vi "Phase_unwrapping2.vi"(10 "Phase at Peaks":dbl[](array[numeric])=[0.5, 1.55, 1.5, -0.641593, 0.358407, 0.358407], 11 "Peak Locations":dbl[](array[numeric])=[0.0, 2.0, 3.0, 4.0]) -> ()   [LabVIEW 2016]
panel:
  out "Array 3":dbl[](array[numeric])
  out "Numeric":i32
  out "Phase out":dbl[](array[numeric])
  out "Boolean":bool
  out "Array 2":dbl[](array[numeric])
  out "Numeric 2":i32
  out "Array":dbl[](array[numeric])
  out "element":i32
  out "Missing Peaks":i32[](array[numeric])=[3, 4, 7, 8, 9]
  in  "Width":dbl=0.02 format="%#_13g"
  in  "Average Spacing":dbl=1.0 format="%#_13g"
  in  "Approximate Phase Difference":dbl=0.5 format="%#_13g"
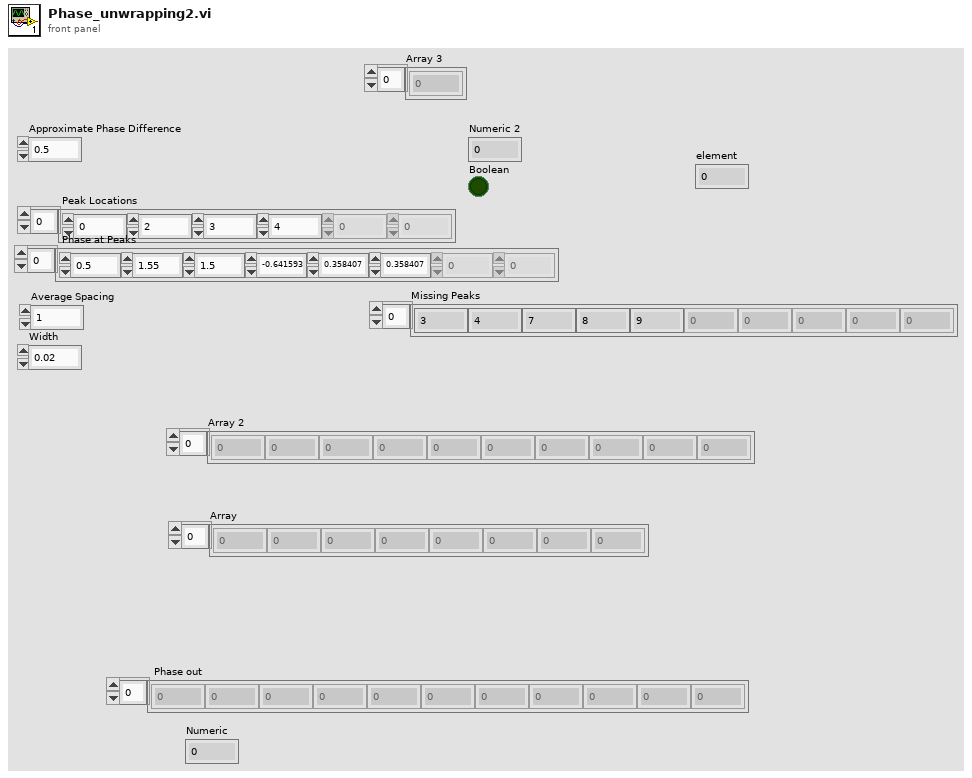
[diagram p1: front panel]
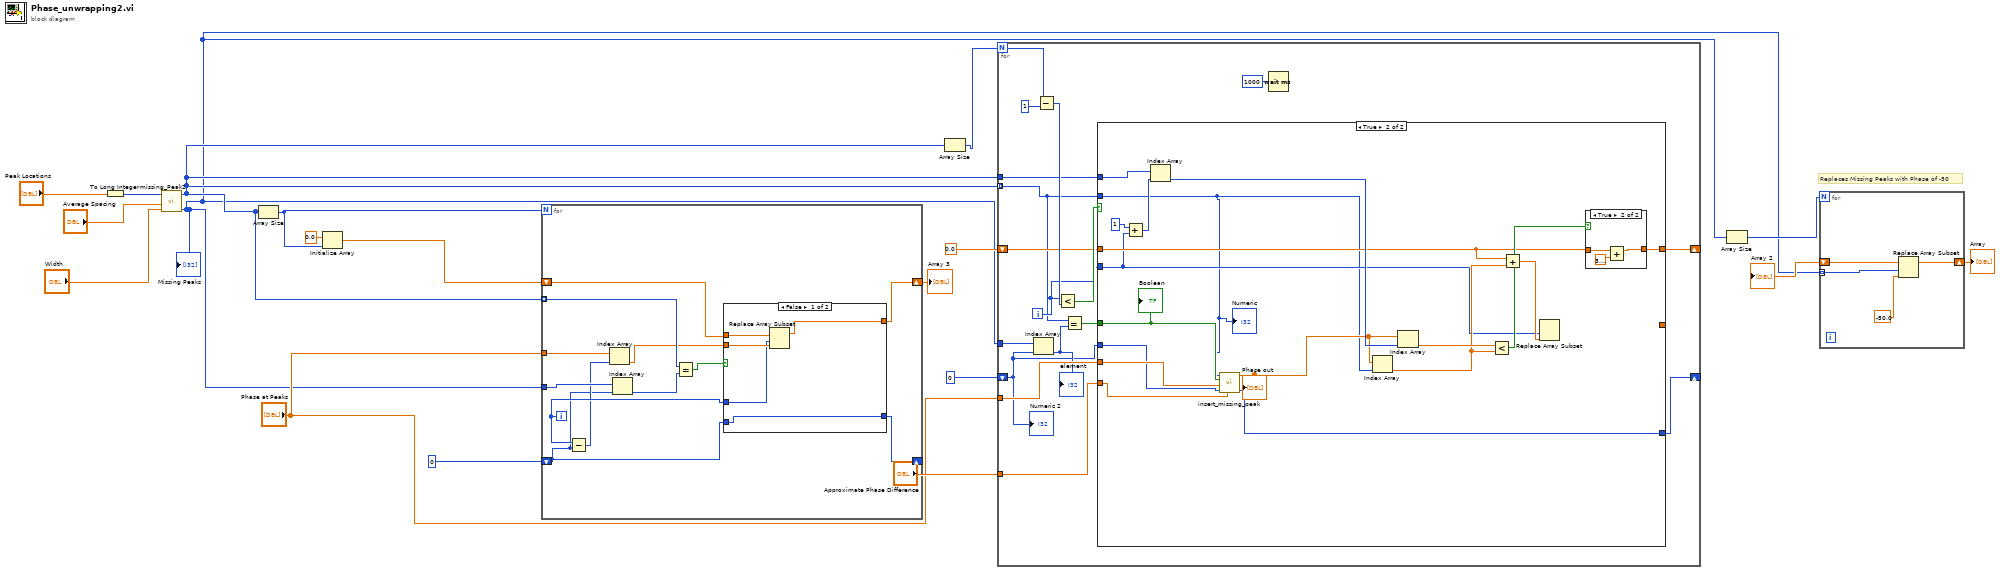
[diagram p0: block diagram]
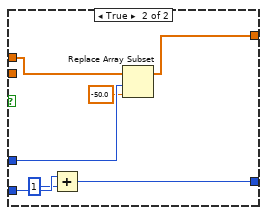
[diagram p2: hidden frame]
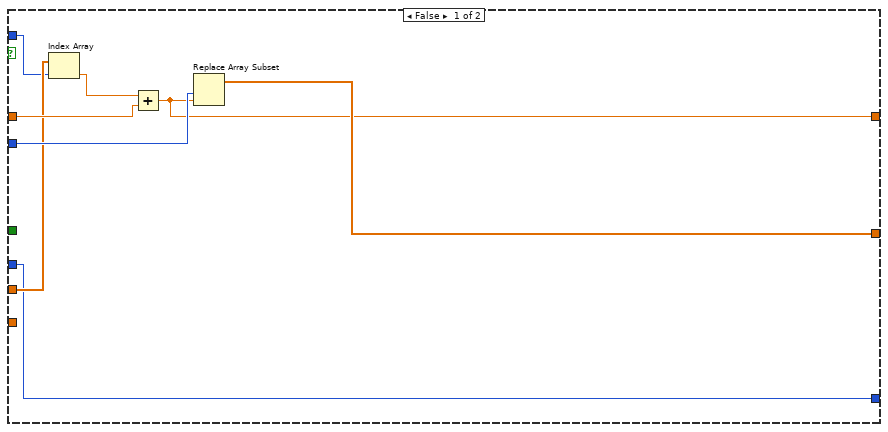
[diagram p3: hidden frame]
diagram:
  # "Replaces Missing Peaks with Phase of -50"
  n1 = To Long Integer(number="Peak Locations") -> (32bit integer=w16:i32[])
  n2 = call "missing_Peak2.vi"("Width"="Width", "Average Spacing"="Average Spacing", 11:w16) -> ("Missing Peaks"=w3:i32[], "Padded Peak Locations"=w4:i32[])  [unwired: 7 in]
  "Missing Peaks" <- w3
  n3 = Array Size(array=w4) -> (size(s)=w7:i32)
  n4 = Initialize Array(0.0 ("element"), w7) -> (w6:dbl[])
  n5 = for {
    N: w7 -> [_]
    shift-right: [w23] -> w1
    shift-left: w6 -> [w26]
    tunnel: w4 -> [w28] mode=indexing
    shift-right: [w20] -> _
    shift-left: 0 -> [w21]
    tunnel: "Phase at Peaks" -> [w31]
    tunnel: w3 -> [w30]
    i -> [w24]
    n6 = Subtract(x=w24, y=w21) -> (x-y=w22:i32)
    n7 = Index Array(array=w31, index=w22) -> (element=w25:dbl)
    n8 = Index Array(array=w30, index=w21) -> (element=w29:i32)
    n9 = Equal?(x=w28, y=w29) -> (x = y?=w27:bool)
    n10 = case shown="False" w27 {
      tunnel: w26 -> [w36 w42]
      tunnel: w25 -> [w35 _]
      tunnel: w24 -> [w34 w41]
      tunnel: [w33 w43] -> w23
      tunnel: w21 -> [w32 w39]
      tunnel: [w32 w37] -> w20
      frame False {
        n11 = Replace Array Subset(array=w36, new element=w35, index=w34) -> (w33:dbl[])
      }
      frame True {
        n12 = Add(x=w39, y=1) -> (x+y=w37:i32)
        n13 = Replace Array Subset(array=w42, new element=-50.0 ("new element/subarray"), index=w41) -> (w43:dbl[])
      }
    }
  }
  "Array 3" <- w1
  n14 = Array Size(array=w4) -> (size(s)=w19:i32)
  n15 = for {
    N: w19 -> [w60]
    tunnel: w4 -> [w50] mode=indexing
    tunnel: w4 -> [w55]
    tunnel: "Phase at Peaks" -> [w54]
    shift-right: [w48] -> _
    shift-left: 0.0 -> [w53]
    tunnel: w3 -> [w51]
    tunnel: "Approximate Phase Difference" -> [w47]
    shift-right: [w45] -> _
    shift-left: 0 -> [w44]
    i -> [w56]
    n16 = Index Array(array=w51, index=w44) -> (element=w46:i32)
    "element" <- w46
    n17 = Subtract(x=w60, y=1) -> (x-y=w58:i32)
    n18 = Less?(x=w56, y=w58) -> (x < y?=w57:bool)
    n19 = Equal?(x=w50, y=w46) -> (x = y?=w49:bool)
    n20 = case shown="True" w57 {
      tunnel: w53 -> [w66 w78]
      tunnel: w56 -> [w68 w73]
      tunnel: [w67 _] -> _
      tunnel: w55 -> [_ w86]
      tunnel: w50 -> [w63 w69]
      tunnel: w54 -> [w64 w76]
      tunnel: [w65 w79] -> w48
      tunnel: w49 -> [_ w75]
      tunnel: w47 -> [_ w74]
      tunnel: w44 -> [w61 w72]
      tunnel: [w61 w71] -> w45
      frame False {
        n21 = Index Array(array=w64, index=w63) -> (element=w62:dbl)
        n22 = Add(x=w62, y=w66) -> (x+y=w65:dbl)
        n23 = Replace Array Subset(new element=w65, index=w68) -> (w67:dbl[])  [unwired: 1 in]
      }
      frame True {
        n24 = Add(x=1, y=w73) -> (x+y=w84:i32)
        n25 = Index Array(array=w86, index=w84) -> (element=w83:i32)
        n26 = call "insert_missing_peak.vi"("Approximate Phase Difference"=w74, "missing peak index in"=w72, "Phase in"=w76, "Boolean"=w75, "Numeric"=w69) -> ("missing peak index out"=w71:i32, "Phase out"=w70:dbl[])  [unwired: 5 in]
        "Phase out" <- w70
        n27 = Index Array(array=w70, index=w69) -> (element=w77:dbl)
        n28 = Index Array(array=w70, index=w83) -> (element=w82:dbl)
        n29 = Less?(x=w82, y=w77) -> (x < y?=w81:bool)
        n30 = Add(x=w78, y=w77) -> (x+y=w80:dbl)
        n31 = Replace Array Subset(new element=w80, index=w73) -> ()  [unwired: 1 in, 1 out]
        n32 = case shown="True" w81 {
          tunnel: w78 -> [w87 w90]
          tunnel: [w87 w88] -> w79
          frame False {
          }
          frame True {
            n33 = Add(x=w90, y=3.141592653589793) -> (x+y=w88:dbl)
          }
        }
        "Boolean" <- w75
        "Numeric" <- w69
      }
    }
    n34 = Wait (ms)(milliseconds to wait=u32 1000) -> ()  [unwired: 1 out]
    "Numeric 2" <- w44
  }
  n35 = Array Size(array=w3) -> (size(s)=w10:i32)
  n36 = for {
    N: w10 -> [_]
    shift-right: [w91] -> w9
    shift-left: [w94] -> w11
    tunnel: w3 -> [w92] mode=indexing
    n37 = Replace Array Subset(array=w94, new element=-50.0 ("new element/subarray"), index=w92) -> (w91:dbl[])
  }
  "Array" <- w9
  "Array 2" <- w11
